vi "U64 to msgpack.vi"(11 "U64":u64) -> (3 "msgpack":u8[](array[numeric]))   [LabVIEW 2020, in "wamplv.lvlib" / "MessagePack.lvclass"]
uses:
  Format bytes.ctl
  MessagePack.lvclass
  MessagePack.lvclass/MessagePack.ctl
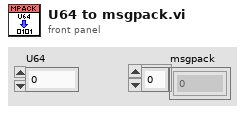
[diagram p1: front panel]
types:
  T1 = typedef "wamplv.lvlib/MessagePack.lvclass/Format bytes.ctl" = u8
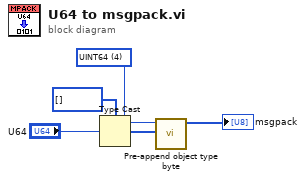
[diagram p0: block diagram]
diagram:
  w5 = T1 4 items=["nil", "UINT8", "UINT16", "UINT32", "UINT64", "INT8", "INT16", "INT32", "INT64"] ("Format byte")
  n1 = Type Cast(type=u8[] [] ("bytes"), x="U64") -> (*(type *) &x=w4:u8[])
  n2 = call "Pre-append object type byte.vi"("data in"=w4, "Format byte"=w5) -> ("bytes add"=→"msgpack":u8[])  [unwired: 9 in]
